vi "Init Jag - Potentiometer Position.vi"(1 "Limit Voltage?":bool, 2 "Jag Refnum Name":string, 3 "D":dbl, 4 "I":dbl, 5 "P":dbl, 6 "Jag ID":i8) -> (0 "MotorControlDevRef":T1={"DeviceStatus"={"status"=FALSE, "code"=0, "source"=""}, "Type"=enum."PWM", "PWM"={"Digital Module"=enum."Digital Module 1", "PWM Channel"=enum."Invalid", "DeadBand"={"Name"="", "maxPositivePwm"=0, "minPositivePwm"=0, "centerPwm"=0, "maxNegativePwm"=0, "minNegativePwm"=0, "angularRange"=0}}, "CAN"={"Device Number"=0, "Control Mode"=enum."Percent VBus", "Semaphore"=refnum, "Max Vout"=12.0}, "Invert"=FALSE, "TransformRef"=refnum, "InvTransformRef"=refnum})   [LabVIEW 2011]
uses:
  <vilib>/Rock Robotics/WPI/MotorControl/WPI_MotorControlDeviceRef.ctl
  <vilib>/Rock Robotics/SystemInterfaces/Typedef/FPGA_TypedefDigitalModule.ctl
  <vilib>/Rock Robotics/SystemInterfaces/DIO/FPGA_DIOPWMChannel.ctl
  <vilib>/Rock Robotics/WPI/PWM/WPI_PWMDeadband.ctl
  <vilib>/Rock Robotics/WPI/CAN/Jaguar/SubVIs/WPI_CANJaguar_ControlMode.ctl
  <vilib>/Rock Robotics/WPI/PWM/WPI_PWMTransform_ConPane.ctl
  <vilib>/Rock Robotics/WPI/CAN/Jaguar/SubVIs/WPI_CANJaguar_PositionReference.ctl
  <vilib>/Rock Robotics/WPI/MotorControl/WPI_MotorControlOpenCANJaguar.vi
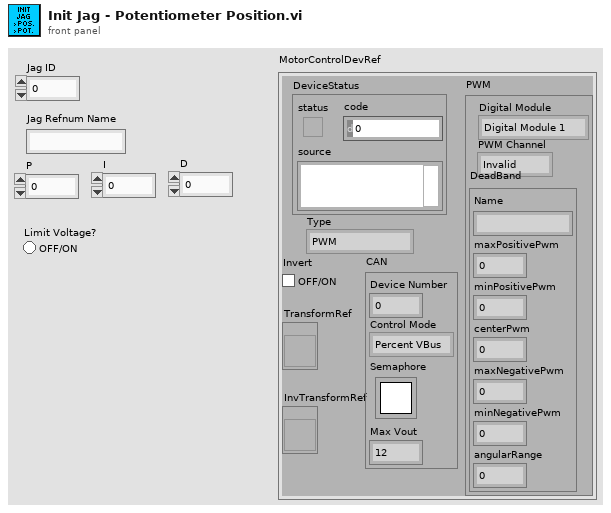
[diagram p1: front panel]
types:
  T1 = typedef "WPI_MotorControlDeviceRef.ctl" = cluster{"DeviceStatus":errorcluster, "Type":enum16{"PWM", "CAN"}, "PWM":cluster{"Digital Module":T2, "PWM Channel":T3, "DeadBand":T4}, "CAN":cluster{"Device Number":u8, "Control Mode":T5, "Semaphore":T6, "Max Vout":dbl}, "Invert":bool, "TransformRef":T7, "InvTransformRef":T7}
  T2 = typedef "FPGA_TypedefDigitalModule.ctl" = enum16{"Digital Module 1", "Digital Module 2"}
  T3 = typedef "FPGA_DIOPWMChannel.ctl" = enum8{"PWM 1", "PWM 2", "PWM 3", "PWM 4", "PWM 5", "PWM 6", "PWM 7", "PWM 8", "PWM 9", "PWM 10", "Invalid"}
  T4 = typedef "WPI_PWMDeadband.ctl" = cluster{"Name":string, "maxPositivePwm":i32, "minPositivePwm":i32, "centerPwm":i32, "maxNegativePwm":i32, "minNegativePwm":i32, "angularRange":u16}
  T5 = typedef "WPI_CANJaguar_ControlMode.ctl" = enum8{"Percent VBus", "Current", "Speed", "Position", "Voltage"}
  T6 = typedef "Semaphore RefNum" = refnum<k1>
  T7 = typedef "WPI_PWMTransform_ConPane.ctl" = refnum<vi>
  T8 = typedef "WPI_CANJaguar_PositionReference.ctl" = u8
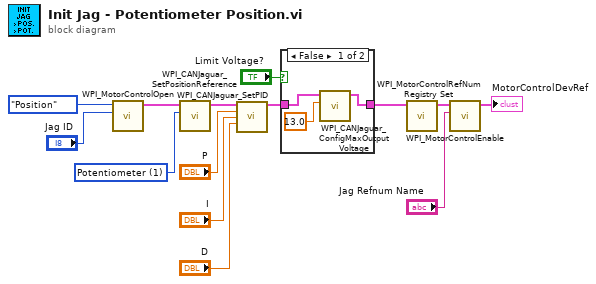
[diagram p0: block diagram]
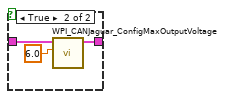
[diagram p2: hidden frame]
diagram:
  w12 = T8 1 items=["Quad Encoder"=0, "Potentiometer"=1, "None"=255] ("Position Reference")
  n1 = call-poly <vilib>:"WPI_MotorControlOpen.vi"("Device Number"="Jag ID", "Control Mode"=WPI_CANJaguar_ControlMode."Position") -> ("MotorControlDeviceRef"=w11:T1)  [unwired: 8 in, 1 out]
  n2 = call <vilib>:"WPI_CANJaguar_SetPositionReference.vi"("Position Reference"=w12, "CAN Jaguar Ref"=w11) -> ("CAN Jaguar Ref Out"=w10:T1)  [unwired: 8 in, 1 out]
  n3 = call <vilib>:"WPI_CANJaguar_SetPID.vi"("CAN Jaguar Ref"=w10, "P"="P", "I"="I", "D"="D") -> ("CAN Jaguar Ref Out"=w3:T1)  [unwired: 10 in, 1 out]
  n4 = case shown="False" "Limit Voltage?" {
    tunnel: w3 -> [w16 w20]
    tunnel: [w15 w19] -> w2
    frame False {
      n5 = call <vilib>:"WPI_CANJaguar_ConfigMaxOutputVoltage.vi"("Maximum Output Voltage"=13.0, "CAN Jaguar Ref"=w16) -> ("CAN Jaguar Ref Out"=w15:T1)  [unwired: 8 in, 1 out]
    }
    frame True {
      n6 = call <vilib>:"WPI_CANJaguar_ConfigMaxOutputVoltage.vi"("Maximum Output Voltage"=6.0, "CAN Jaguar Ref"=w20) -> ("CAN Jaguar Ref Out"=w19:T1)  [unwired: 8 in, 1 out]
    }
  }
  n7 = call <vilib>:"WPI_MotorControlEnable.vi"("CAN Jaguar Ref"=w2) -> ("CAN Jaguar Ref Out"=w6:T1)  [unwired: 9 in, 1 out]
  n8 = call <vilib>:"WPI_MotorControlRefNum Registry Set.vi"("refnum name"="Jag Refnum Name", "MotorControlDevRef"=w6) -> ("MotorControlDevRef"=→"MotorControlDevRef":T1)  [unwired: 8 in, 1 out]
